vi "Measurement_Zshape.vi"() -> ()   [LabVIEW 2016]
uses:
  Control/Coordinate.ctl
  <vilib>/Instr/_visa.llb/VISA Flush IO Buffer Mask.ctl
  <vilib>/Instr/_visa.llb/VISA Configure Serial Port (Instr).vi
panel:
  in  "File Name":string
  in  "Point1(ref)":T1={"X"=968.59881, "Y"=892.69941, "Z"=0.0, "U"=0.0} {"U" format="%#.5g"; "X" format="%#.5g"; "Y" format="%#.5g"; "Z" format="%#.5g"}
  out "B":bool=TRUE
  in  "VISA resource name":refnum<visa-resource-name>="COM4"
  in  "flow control":u16(ring) items=["None"=0, "XON/XOFF"=1, "RTS/CTS"=2, "DTR/DSR"=4]
  in  "stop bits":u16(ring)=10 items=["1"=10, "1.5"=15, "2.0"=20]
  in  "parity":u16(ring)=2 items=["None", "Odd", "Even", "Mark", "Space"]
  in  "data bits":u16=8 min=5 max=8 step=1
  in  "baud rate":u32=1500000
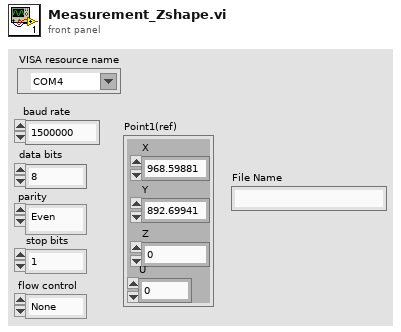
[diagram p1: front panel]
types:
  T1 = typedef "Coordinate.ctl" = cluster{"X":dbl, "Y":dbl, "Z":dbl, "U":dbl}
  T2 = typedef "VISA Flush IO Buffer Mask.ctl" = u16
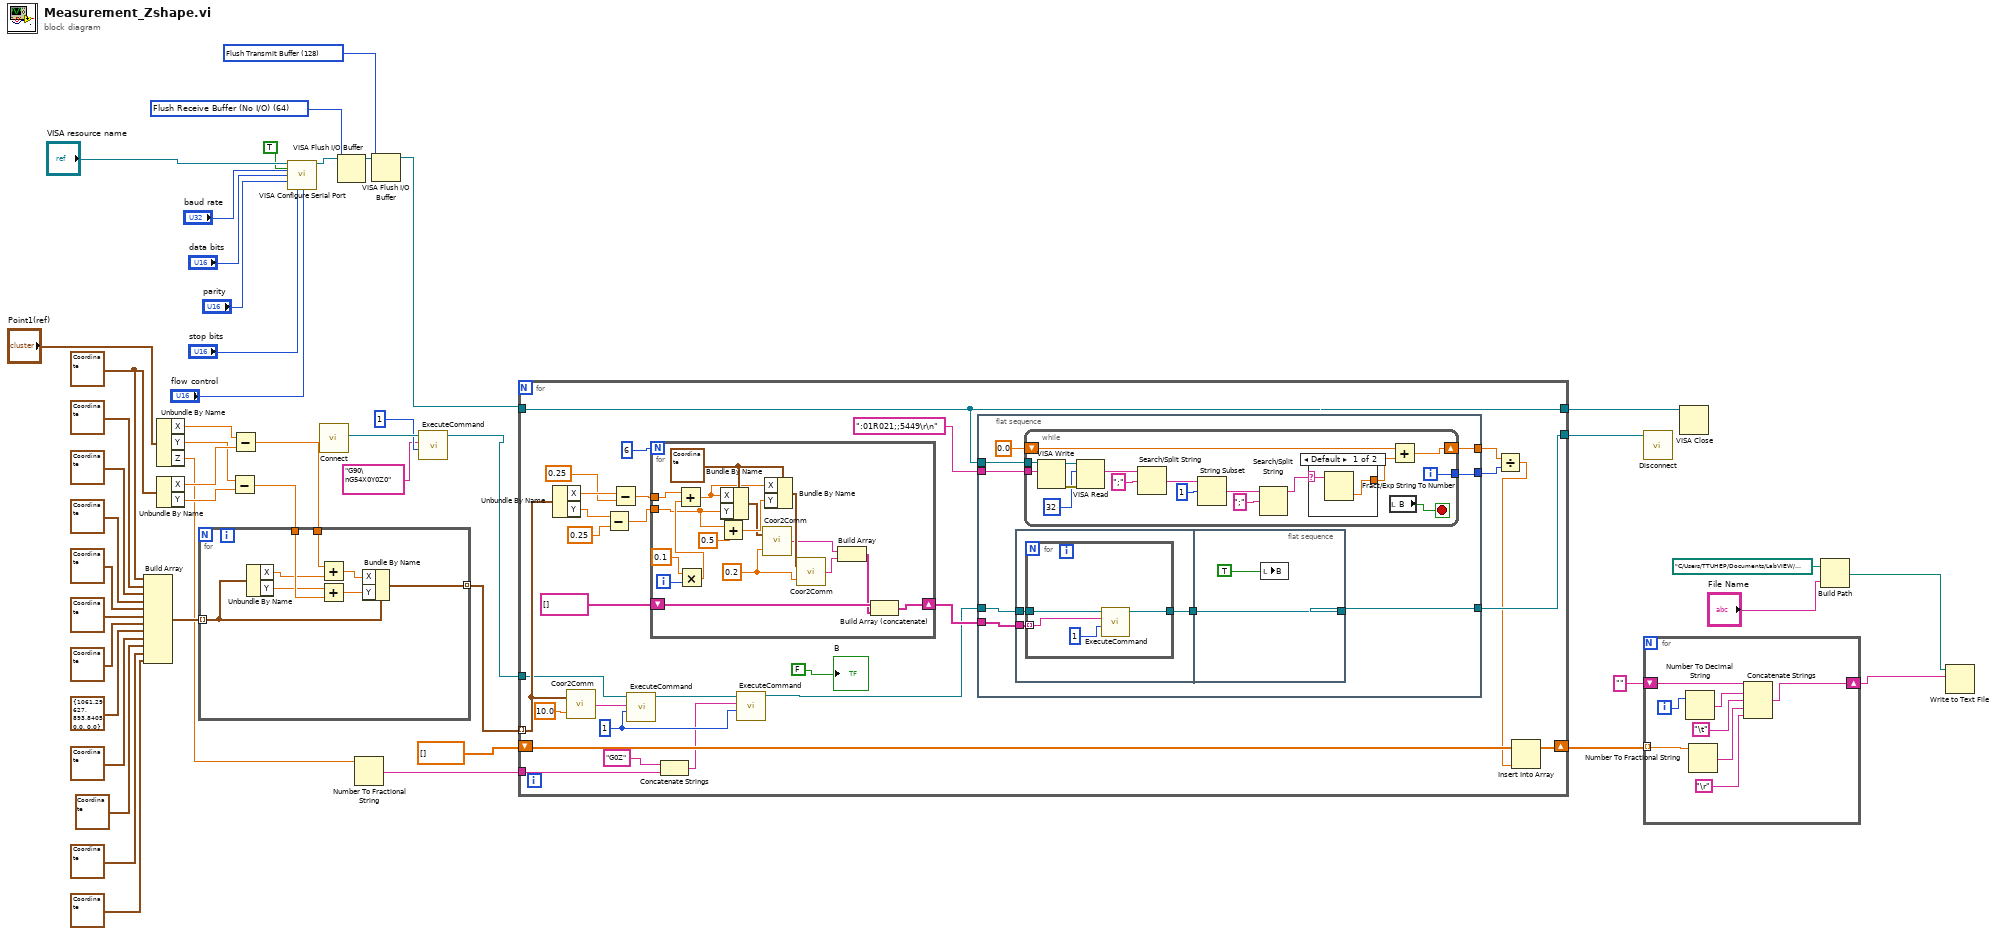
[diagram p0: block diagram]
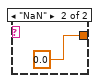
[diagram p2: hidden frame]
diagram:
  w9 = T2 128 items=["Flush Receive Buffer"=16, "Write Transmit Buffer to Device"=32, "Flush Receive Buffer (No I/O)"=64, "Flush Transmit Buffer"=128] ("Mask")
  w10 = T2 64 items=["Flush Receive Buffer"=16, "Write Transmit Buffer to Device"=32, "Flush Receive Buffer (No I/O)"=64, "Flush Transmit Buffer"=128] ("Mask")
  w25 = T1 {"X"=968.59881, "Y"=892.69941, "Z"=0.0, "U"=0.0} ("Cluster")
  n1 = Build Array(w25, T1 {"X"=935.82847, "Y"=892.39476, "Z"=0.0, "U"=0.0} ("Cluster"), T1 {"X"=984.00934, "Y"=920.23702, "Z"=0.0, "U"=0.0} ("Cluster"), T1 {"X"=968.4175, "Y"=946.44696, "Z"=0.0, "U"=0.0} ("Cluster"), T1 {"X"=1015.22496, "Y"=920.85666, "Z"=0.0, "U"=0.0} ("Cluster"), T1 {"X"=1029.74858, "Y"=946.23572, "Z"=0.0, "U"=0.0} ("Cluster"), T1 {"X"=1032.16519, "Y"=893.82319, "Z"=0.0, "U"=0.0} ("Cluster"), T1 {"X"=1061.29627, "Y"=893.8405, "Z"=0.0, "U"=0.0} ("Cluster"), T1 {"X"=1015.70805, "Y"=866.10244, "Z"=0.0, "U"=0.0} ("Cluster"), T1 {"X"=1031.05463, "Y"=839.92674, "Z"=0.0, "U"=0.0} ("Cluster"), T1 {"X"=984.40385, "Y"=865.83641, "Z"=0.0, "U"=0.0} ("Cluster"), T1 {"X"=969.65826, "Y"=840.13643, "Z"=0.0, "U"=0.0} ("Cluster")) -> (w27:T1[])
  n2 = Unbundle By Name("Point1(ref)") -> ("X"=w24:dbl, "Y"=w22:dbl, "Z"=w17:dbl)
  n3 = Unbundle By Name(w25) -> ("X"=w23:dbl, "Y"=w21:dbl)
  n4 = Subtract(x=w22, y=w21) -> (x-y=w19:dbl)
  n5 = Subtract(x=w24, y=w23) -> (x-y=w20:dbl)
  n6 = for {
    tunnel: w27 -> [w56] mode=indexing
    tunnel: w20 -> [w53]
    tunnel: w19 -> [w52]
    tunnel: [w49] -> w16 mode=indexing
    n7 = Unbundle By Name(w56) -> ("X"=w50:dbl, "Y"=w51:dbl)
    n8 = Add(x=w53, y=w50) -> (x+y=w54:dbl)
    n9 = Add(x=w51, y=w52) -> (x+y=w55:dbl)
    n10 = Bundle By Name(cluster=w56, "X"=w54, "Y"=w55) -> (w49:T1)
  }
  n11 = call-poly "VISA Configure Serial Port"("VISA resource name"="VISA resource name", "Enable Termination\nChar (T)"=TRUE, "baud rate (9600)"="baud rate", "data bits (8)"="data bits", "parity (0:none)"="parity", "stop bits (10: 1 bit)"="stop bits", "flow control (0:none)"="flow control") -> ("VISA resource name out"=w12:refnum<visa-resource-name>)  [unwired: 7 in, 1 out]
  n12 = call "Connect.vi"() -> ("controller"=w4:refnum<k24>)  [unwired: 10 in, 1 out]
  n13 = VISA Flush I/O Buffer(VISA resource name=w12, mask (16)=w10) -> (VISA resource name out=w11:refnum<visa-resource-name>)  [unwired: 1 in, 1 out]
  n14 = Number To Fractional String(number=w17) -> (F-format string=w18:string)  [unwired: 3 in]
  n15 = VISA Flush I/O Buffer(VISA resource name=w11, mask (16)=w9) -> (VISA resource name out=w8:refnum<visa-resource-name>)  [unwired: 1 in, 1 out]
  n16 = call "ExecuteCommand.vi"("taskId"=1, "Command Code"="G90\nG54X0Y0Z0", "controller in"=w4) -> ("controller out"=w2:refnum<k24>)  [unwired: 6 in, 2 out]
  n17 = for {
    tunnel: w16 -> [w83] mode=indexing
    shift-right: [w66] -> w15
    shift-left: dbl[] [] ("Array") -> [w65]
    tunnel: w2 -> [w74]
    tunnel: [w72] -> w29
    tunnel: w8 -> [w70]
    tunnel: [w70] -> w28
    tunnel: w18 -> [w60]
    w61 = 1
    n18 = Unbundle By Name(w83) -> ("X"=w82:dbl, "Y"=w78:dbl)
    n19 = call "Coor2Comm.vi"("Numeric"=10.0, "Cluster"=w83) -> ("String"=w57:string)
    n20 = Subtract(x=w78, y=0.25) -> (x-y=w79:dbl)
    n21 = Subtract(x=w82, y=0.25) -> (x-y=w80:dbl)
    n22 = call "ExecuteCommand.vi"("taskId"=w61, "Command Code"=w57, "controller in"=w74) -> ("controller out"=w62:refnum<k24>)  [unwired: 6 in, 2 out]
    n23 = for {
      N: 6 -> [_]
      tunnel: w80 -> [w137]
      tunnel: w79 -> [w132]
      shift-right: [w128] -> w73
      shift-left: string[] [] -> [w129]
      i -> [w139]
      w123 = 0.2
      w135 = T1 {"X"=1026.02948, "Y"=917.39243, "Z"=0.0, "U"=0.0} ("Cluster")
      n24 = Multiply(x=0.1, y=w139) -> (x*y=w136:dbl)
      n25 = Add(x=w137, y=w136) -> (x+y=w134:dbl)
      n26 = Add(x=w132, y=0.5) -> (x+y=w133:dbl)
      n27 = Bundle By Name(cluster=w135, "X"=w134, "Y"=w132) -> (w130:T1)
      n28 = call "Coor2Comm.vi"("Numeric"=w123, "Cluster"=w130) -> ("String"=w125:string)
      n29 = Bundle By Name(cluster=w135, "X"=w134, "Y"=w133) -> (w127:T1)
      n30 = call "Coor2Comm.vi"("Numeric"=w123, "Cluster"=w127) -> ("String"=w126:string)
      n31 = Build Array(w125, w126) -> (w124:string[])
      n32 = Build Array (concatenate)(w129, w124) -> (w128:string[])
    }
    n33 = Concatenate Strings("G0Z", w60) -> (w58:string)
    n34 = call "ExecuteCommand.vi"("taskId"=w61, "Command Code"=w58, "controller in"=w62) -> ("controller out"=w63:refnum<k24>)  [unwired: 6 in, 2 out]
    n35 = flat-sequence {
      tunnel: w63 -> [w93]
      tunnel: w73 -> [w92]
      tunnel: [w91] -> w72
      tunnel: ":01R021;;5449\r\n" ("Command") -> [w90]
      tunnel: w70 -> [w89]
      tunnel: [w87] -> w67
      tunnel: [w85] -> w68
      frame #0 {
        n36 = flat-sequence {
          tunnel: w93 -> [w96]
          tunnel: w92 -> [w95]
          tunnel: [w94] -> w88
          tunnel: [w102] -> w91
          tunnel: w88 -> [w102]
          frame #0 {
            n37 = for {
              tunnel: w96 -> [w100]
              tunnel: w95 -> [w99] mode=indexing
              tunnel: [w98] -> w94
              n38 = call "ExecuteCommand.vi"("taskId"=1, "Command Code"=w99, "controller in"=w100) -> ("controller out"=w98:refnum<k24>)  [unwired: 6 in, 2 out]
            }
          }
          frame #1 {
            n39 = local write "B"(TRUE) -> ()
          }
        }
        n40 = while {
          tunnel: w90 -> [w117]
          tunnel: w89 -> [w116]
          tunnel: [w107] -> w87
          shift-right: [w106] -> w85
          shift-left: 0.0 -> [w105]
          i -> [w107]
          stop <- w108 stop-if-true
          n41 = VISA Write(VISA resource name=w116, write buffer=w117) -> (VISA resource name out=w119:refnum<visa-resource-name>, error out=w118:errorcluster)  [unwired: 1 in, 1 out]
          n42 = VISA Read(VISA resource name=w119, byte count=32, error in (no error)=w118) -> (read buffer=w110:string)  [unwired: 3 out]
          n43 = Search/Split String(string=w110, search string/char (-)=";") -> (match + rest of string=w111:string)  [unwired: 1 in, 2 out]
          n44 = String Subset(string=w111, offset (0)=1) -> (substring=w112:string)  [unwired: 1 in]
          n45 = Search/Split String(string=w112, search string/char (-)=";") -> (substring before match=w109:string)  [unwired: 1 in, 2 out]
          n46 = case shown="Default" w109 {
            selector: w109 -> [w121 _]
            tunnel: [w120 0.0] -> w104
            frame Default {
              n47 = Fract/Exp String To Number(string=w121) -> (number=w120:dbl)  [unwired: 3 in, 1 out]
            }
            frame "NaN" {
            }
          }
          n48 = local read "B"() -> (w108:bool)
          n49 = Add(x=w105, y=w104) -> (x+y=w106:dbl)
        }
      }
    }
    n50 = Divide(x=w68, y=w67) -> (x/y=w64:dbl)
    n51 = Insert Into Array(array=w65, new element=w64) -> (w66:dbl[])  [unwired: 1 in]
    "B" <- FALSE
  }
  n52 = call "Disconnect.vi"("controller"=w29) -> ()  [unwired: 10 in, 1 out]
  n53 = for {
    tunnel: w15 -> [w147] mode=indexing
    shift-right: [w145] -> w13
    shift-left: "" -> [w146]
    i -> [w144]
    n54 = Number To Decimal String(number=w144) -> (decimal integer string=w143:string)  [unwired: 1 in]
    n55 = Number To Fractional String(number=w147) -> (F-format string=w141:string)  [unwired: 3 in]
    n56 = Concatenate Strings(w146, w143, "\t", w141, "\r") -> (w145:string)
  }
  n57 = VISA Close(VISA resource name=w28) -> ()  [unwired: 1 in, 1 out]
  n58 = Build Path(base path=path "C:/Users/TTUHEP/Documents/LabVIEW/Data/Center", name or relative path="File Name") -> (appended path=w5:path)
  n59 = Write to Text File(file (use dialog)=w5, text=w13) -> ()  [unwired: 2 in, 3 out]
